vi "Is String Found In Lib Tokens.vi"(10 "String":string, 11 "Config":refnum<class "TAF Proj Config.lvclass">) -> (3 "Not Found?":bool)   [LabVIEW 2021, in "TAF Proj Document Type.lvlib" / "Project Parser.lvlib"]
uses:
  <vilib>/Wovalab/AntiDoc/Document Type/Add-ons/LabVIEW TAF Project/Project Parser/Project Parser.lvlib
  <vilib>/Wovalab/AntiDoc/Document Type/Add-ons/LabVIEW TAF Project/TAF Proj Config/TAF Proj Config.lvclass
  <vilib>/Wovalab/AntiDoc/Document Type/Add-ons/LabVIEW TAF Project/TAF Proj Config/TAF Proj Config.lvclass/TAF Proj Config.ctl
  <vilib>/Wovalab/AntiDoc/Document Type/Add-ons/LabVIEW TAF Project/TAF Proj Config/Read Lib Tokens.vi
  <vilib>/regexp/Match Regular Expression.xnode
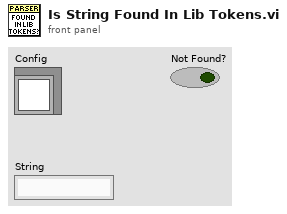
[diagram p1: front panel]
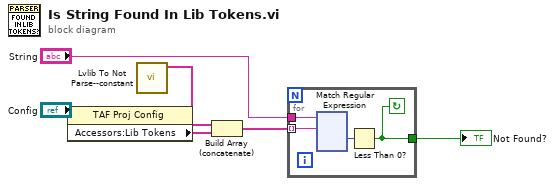
[diagram p0: block diagram]
diagram:
  n1 = property class="TAF Proj Config"(reference="Config") -> ("Accessors:Lib Tokens"=w2:string[])  [unwired: 1 in, 2 out]
  n2 = call <vilib>:"Lvlib To Not Parse--constant.vi"() -> ("Lvlib Name"=w3:string[])  [unwired: 11 in]
  n3 = Build Array (concatenate)(w3, w2) -> (w1:string[])
  n4 = for {
    tunnel: "String" -> [w9]
    tunnel: [w7] -> w6
    tunnel: w1 -> [w10] mode=indexing
    stop <- w7 continue-if-true
    n5 = xnode "Match Regular Expression"("input string"=w9, "regular expression"=w10) -> ("offset past match"=w8:i32)  [unwired: 4 in, 4 out]
    n6 = Less Than 0?(x=w8) -> (x < 0?=w7:bool)
  }
  "Not Found?" <- w6
